vi "Check All DAQ Stopped.vi"(8 "error in (no error)":errorcluster, 11 "Cfg Grandmaster in":refnum<class "Cfg Grandmaster.lvclass">) -> (0 "error out":errorcluster, 3 "Cfg Grandmaster out":refnum<class "Cfg Grandmaster.lvclass">)   [LabVIEW 2012, in "Configuration Grandmaster.lvlib" / "Cfg Grandmaster.lvclass"]
uses:
  Cfg Grandmaster.lvclass
  Cfg Grandmaster.lvclass/Cfg Grandmaster.ctl
  Common/Controls/DAQMan Mode.ctl
  <vilib>/ActorFramework/Time-Delayed Send Message/Time-Delay Override Options.ctl
  Class FP Ctrls/FP Controls.lvclass
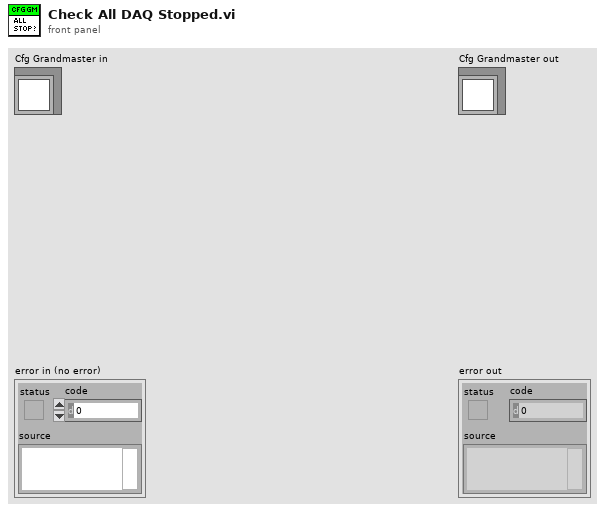
[diagram p1: front panel]
types:
  T1 = typedef "Time-Delay Override Options.ctl" = enum16{"Send next copy now", "Skip next scheduled copy", "Send next copy now and stop all further copies", "Stop all further copies"}
  T2 = typedef "DAQMan Mode.ctl" = enum16{"Cfg", "Run", "Shutting Down"}
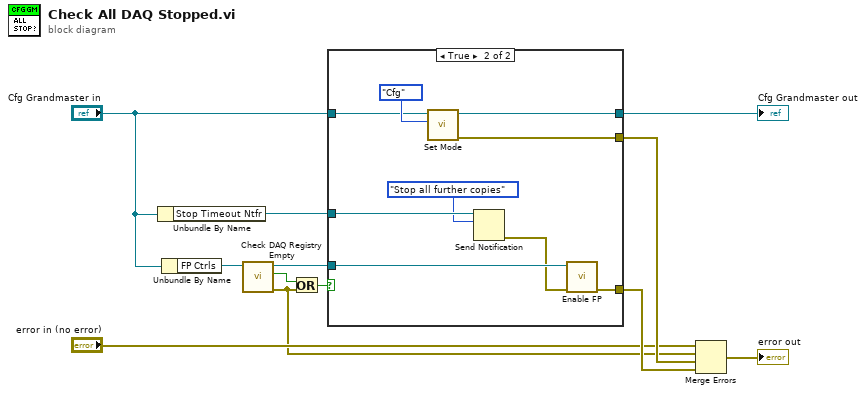
[diagram p0: block diagram]
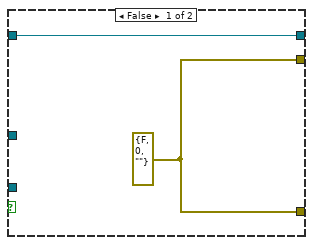
[diagram p2: hidden frame]
diagram:
  n1 = Unbundle By Name("Cfg Grandmaster in") -> ("Stop Timeout Ntfr"=w6:refnum<notifier>)
  n2 = Unbundle By Name("Cfg Grandmaster in") -> ("FP Ctrls"=w11:refnum<class "FP Controls.lvclass">)
  n3 = call "Check DAQ Registry Empty.vi"("FP Controls in"=w11) -> ("error out"=w1:errorcluster, "DAQ Reg Empty?"=w10:bool, "FP Controls out"=w4:refnum<class "FP Controls.lvclass">)  [unwired: 8 in]
  n4 = Or(x=w10, y=w1) -> (x .or. y?=w9:bool)
  n5 = case shown="True" w9 {
    tunnel: [w14 w20] -> w12
    tunnel: [w13 w19] -> w8
    tunnel: "Cfg Grandmaster in" -> [w14 w21]
    tunnel: w6 -> [_ w23]
    tunnel: w4 -> [_ w17]
    tunnel: [w13 w15] -> w3
    frame False {
      w13 = errorcluster {"status"=FALSE, "code"=0, "source"=""} ("error out")
    }
    frame True {
      n6 = call "Set Mode.vi"("Mode"=DAQMan_Mode."Cfg", "Cfg Grandmaster in"=w21) -> ("error out"=w19:errorcluster, "Cfg Grandmaster out"=w20:refnum<class "Cfg Grandmaster.lvclass">)  [unwired: 8 in]
      n7 = Send Notification(notification=Time-Delay_Override_Options."Stop all further copies", notifier=w23) -> (error out=w16:errorcluster)  [unwired: 1 in, 1 out]
      n8 = call "Enable FP.vi"("error in (no error)"=w16, "FP Controls in"=w17) -> ("error out"=w15:errorcluster)  [unwired: 8 in, 1 out]
    }
  }
  "Cfg Grandmaster out" <- w12
  n9 = Merge Errors("error in (no error)", w1, w8, w3) -> (→"error out":errorcluster)
